vi "Test_WriteValue_LatchingBoolean_Error.vi"(8 "error in (no error)":errorcluster, 11 "TestCase in":refnum<class "TestTerminalSignalingValueBinding.lvclass">) -> (0 "error out":errorcluster, 3 "TestCase out":refnum<class "TestTerminalSignalingValueBinding.lvclass">)   [LabVIEW 2017, in "TestTerminalSignalingValueBinding.lvclass"]
uses:
  TestTerminalSignalingValueBinding.lvclass
  Source/Concrete/TerminalSignalingValueBinding/TerminalSignalingValueBinding.lvclass
  C:/Git/composed-transport/Source/ITransport/ITransport.lvclass
  Source/ITransport/ITransport.lvclass
panel:
  out "Return Error":errorcluster
  in  "OK Button":bool
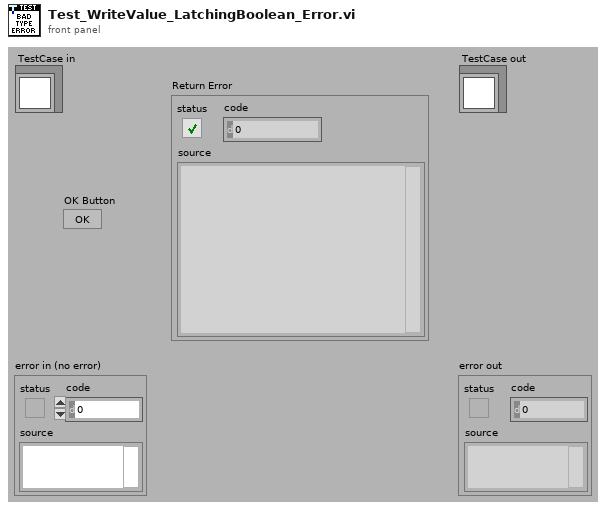
[diagram p1: front panel]
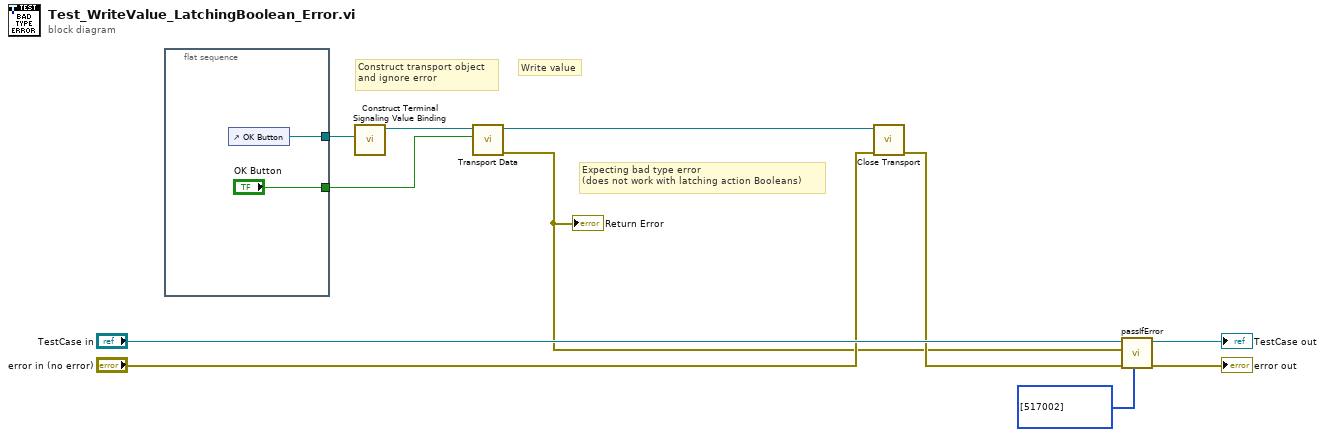
[diagram p0: block diagram]
diagram:
  # "Write value"
  # "Expecting bad type error\n(does not work with latching action Booleans)"
  # "Construct transport object\nand ignore error"
  n1 = flat-sequence {
    tunnel: [w13] -> w7
    tunnel: ["OK Button"] -> w2
    frame #0 {
      n2 = control-ref of="OK Button"() -> (w13:refnum<vi>)
    }
  }
  n3 = call "Construct Terminal Signaling Value Binding.vi"("Ctl Refnum"=w7) -> ("TerminalSignalingValueBinding"=w8:refnum<class "TerminalSignalingValueBinding.lvclass">)  [unwired: 9 in, 1 out]
  n4 = call "Transport Data.vi"("Value"=w2, "ITransport in"=w8) -> ("error out"=w3:errorcluster, "ITransport out"=w4:refnum<class "TerminalSignalingValueBinding.lvclass">)  [unwired: 8 in]
  "Return Error" <- w3
  n5 = call-dynamic "Close Transport.vi"("error in (no error)"="error in (no error)", "ITransport in"=w4) -> ("error out"=w5:errorcluster)  [unwired: 9 in]
  n6 = call-dynamic "passIfError.vi"("passing error codes (default = any error code)"=i32[] [517002], "error in (no error)"=w5, "error"=w3, "TestCase in"="TestCase in") -> ("error out"=→"error out":errorcluster, "TestCase out"=→"TestCase out":refnum<class "TestTerminalSignalingValueBinding.lvclass">)  [unwired: 6 in]
